vi "Pre Launch Init.vi"(11 "Nested in":refnum<class "Function Generator Actor.lvclass">) -> (0 "error out":errorcluster, 3 "Nested out":refnum<class "Function Generator Actor.lvclass">)   [LabVIEW 2020, in "Function Generator Actor.lvlib" / "Function Generator Actor.lvclass"]
doc: "(<B>Filename</B>: Actor Framework.lvlib:Actor.lvclass:Pre Launch Init.vi)\n\nDefines behavior that occurs after the Launch Nested Actor method is invoked but before the actor's Actor Core method begins running.\n\nBy default, this method does nothing. A descendant class may override it to define behavior."
uses:
  Function Generator Actor.lvclass
  Function Generator Actor.lvclass/Function Generator Actor.ctl
  <vilib>/ActorFramework/Actor/Actor.lvclass
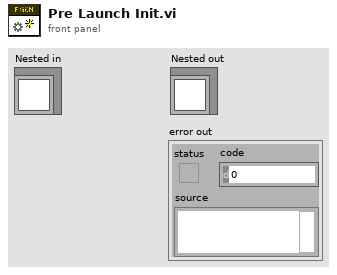
[diagram p1: front panel]
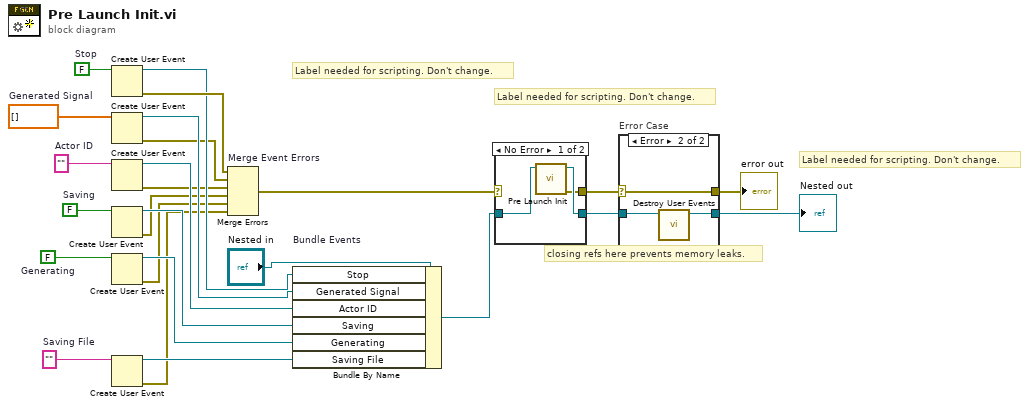
[diagram p0: block diagram]
diagram:
  w3 = ""  # Saving File
  w6 = FALSE  # Generating
  w9 = FALSE  # Saving
  w12 = ""  # Actor ID
  w15 = dbl[] []  # Generated Signal
  w24 = FALSE  # Stop
  # "Label needed for scripting. Don't change."
  # "Label needed for scripting. Don't change."
  # "Label needed for scripting. Don't change."
  # "closing refs here prevents memory leaks."
  n1 = Create User Event(user event datatype=w24) -> (user event=w21:refnum<user-event>, error out=w23:errorcluster)  [unwired: 1 in]
  n2 = Create User Event(user event datatype=w15) -> (user event=w14:refnum<user-event>, error out=w13:errorcluster)  [unwired: 1 in]
  n3 = Create User Event(user event datatype=w12) -> (user event=w11:refnum<user-event>, error out=w10:errorcluster)  [unwired: 1 in]
  n4 = Create User Event(user event datatype=w9) -> (user event=w8:refnum<user-event>, error out=w7:errorcluster)  [unwired: 1 in]
  n5 = Create User Event(user event datatype=w6) -> (user event=w5:refnum<user-event>, error out=w4:errorcluster)  [unwired: 1 in]
  n6 = Create User Event(user event datatype=w3) -> (user event=w2:refnum<user-event>, error out=w1:errorcluster)  [unwired: 1 in]
  n7 = Merge Errors "Merge Event Errors"(w23, w13, w10, w7, w4, w1) -> (w17:errorcluster)
  n8 = Bundle By Name "Bundle Events"(cluster="Nested in", "Stop"=w21, "Generated Signal"=w14, "Actor ID"=w11, "Saving"=w8, "Generating"=w5, "Saving File"=w2) -> (w18:refnum<class "Function Generator Actor.lvclass">)
  n9 = case shown="No Error" w17 {
    selector: w17 -> [_ w30]
    tunnel: [w28 w29] -> w19
    tunnel: w18 -> [w27 w29]
    tunnel: [w26 w30] -> w16
    frame No Error {
      n10 = call-parent "Pre Launch Init.vi"("Actor in"=w27) -> ("error out"=w26:errorcluster, "Actor out"=w28:refnum<class "Function Generator Actor.lvclass">)  [unwired: 9 in]
    }
    frame Error {
    }
  }
  n11 = case "Error Case" shown="Error" w16 {
    selector: w16 -> [w31 w35]
    tunnel: w19 -> [w32 w34]
    tunnel: [w32 w33] -> w22
    tunnel: [w31 w35] -> w20
    frame No Error {
    }
    frame Error {
      n12 = call "Destroy User Events.vi"("UI Template in"=w34) -> ("UI Template out"=w33:refnum<class "Function Generator Actor.lvclass">)  [unwired: 10 in]
    }
  }
  "error out" <- w20
  "Nested out" <- w22
